vi "RTTAutomation.vi"() -> ()   [LabVIEW 2011]
doc: "This application is used to build test scripts for embedded software validation through the design process (MIL, HIL, TestCells)"
uses:
  SubVIs/TS_controls.ctl
  SubVIs/UI_Pages.ctl
  SubVIs/ScriptStepTypeDef.ctl
panel:
  in  "Stop":bool
  in  "Navigation Bar":T1
  in  "TestStand UI ExecutionView Manager":refnum<k7>(container)
  in  "TestStand UI SequenceFileView Manager":refnum<k7>(container)
  in  "Tab Control":T2(tab)
  out "State":string="Ready"
  out "Saved?":bool=TRUE
  in  "Save As Test Script":bool
  in  "Add_Test Procedure":bool
  in  "TreeCtl":string(tree)="System Config"
  in  "Open Test Script":bool
  in  "Save Test Script":bool
  in  "New Test Script":bool
  in  "Run Seq":refnum<k7>(container)
  in  "Open Seq file":refnum<k7>(container)
  in  "Test Sequence Viewer":refnum<k7>(container) caption="TestStand Sequence"
  in  "Generate":bool
  in  "Report Viewer":refnum<k7>(container)
  in  "Open DDreport":bool
  in  "Open TS Report":bool
  in  "Configuration Paths":T3
  out "Missing Files":bool
  in  "TestStand UI Application Manager (in)":refnum<k7>(container)
  # "Real-Time Test Automation"
  # "Test Script Builder"
  # "Sequence Builder"
  # "Report Viewer"
  # "Utilities"
  # "System Configuration"
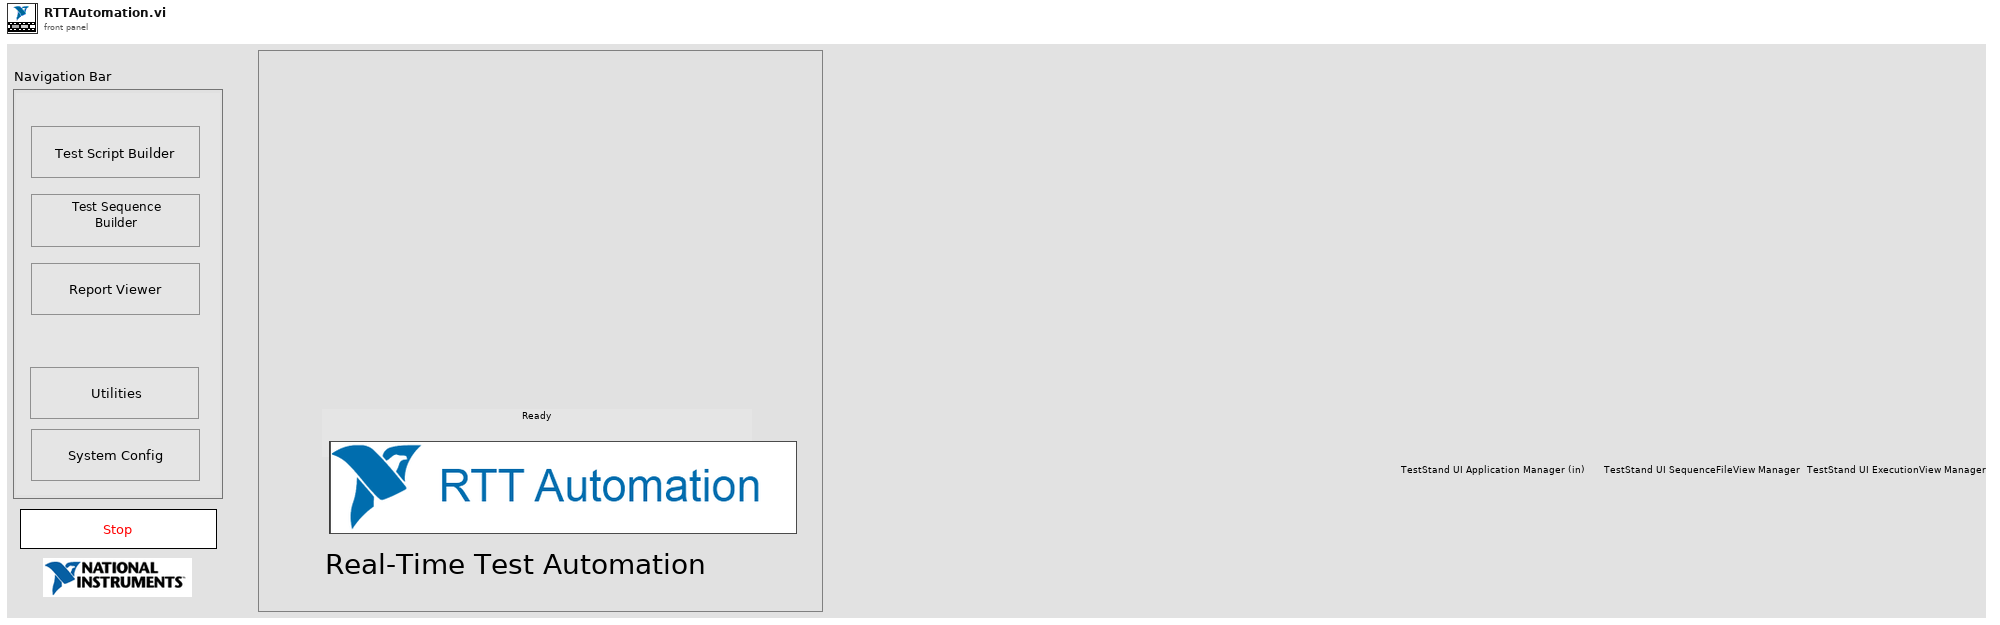
[diagram p1: front panel]
types:
  T1 = cluster{"Script Builder":bool, "Test Sequence Builder":bool, "Report":bool, "Utilities":bool, "System Config":bool}
  T2 = enum32{"Splash", "Test Script Builder", "Sequence Builder", "Report", "Utilities", "System Config"}
  T3 = cluster{"Working Directory":path, "Folder to Requirements Document":path, "Folder to the VeriStand Projects":path, "Folder to Stimuls Profiles":path, "Folder to Calibration files":path, "Folder to Analysis Scripts":path}
  T4 = typedef "ScriptStepTypeDef.ctl" = cluster{"Indent Level":i32, "Tag":string, "Step component":string, "Req":string, "Parent Tag":string, "Symbol Index":i32}
  T5 = enum8{"Enabled", "Disabled", "Disabled and Grayed Out"}
  T6 = typedef "UI_Pages.ctl" = enum32{"Splash", "Test Script Builder", "Sequence Builder", "Report", "Utilities", "System Config"}
  T7 = typedef "TS_controls.ctl" = cluster{"Open Seq file":refnum<k7>, "Test Sequence Viewer":refnum<k7>, "Run Seq":refnum<k7>}
  T8 = typedef "Config cluster.ctl" = cluster{"Working Directory":path, "Folder to Requirements Documents":path, "Folder to VeriStand Project files":path, "Folder to Stimuls Profiles":path, "Folder to Calibration files":path, "Folder to Analysis Scripts":path, "Requirements":string[], "Tree Control":refnum<vi>, "vi reference":refnum<vi>}
  T9 = typedef "LVPoint32TypeDef.ctl" = cluster{"Horizontal":i32, "Vertical":i32}
  T10 = enum32{"invalid app kind", "Development System", "Run Time System", "Student Edition", "Embedded LabVIEW", "Evaluation", "Custom"}
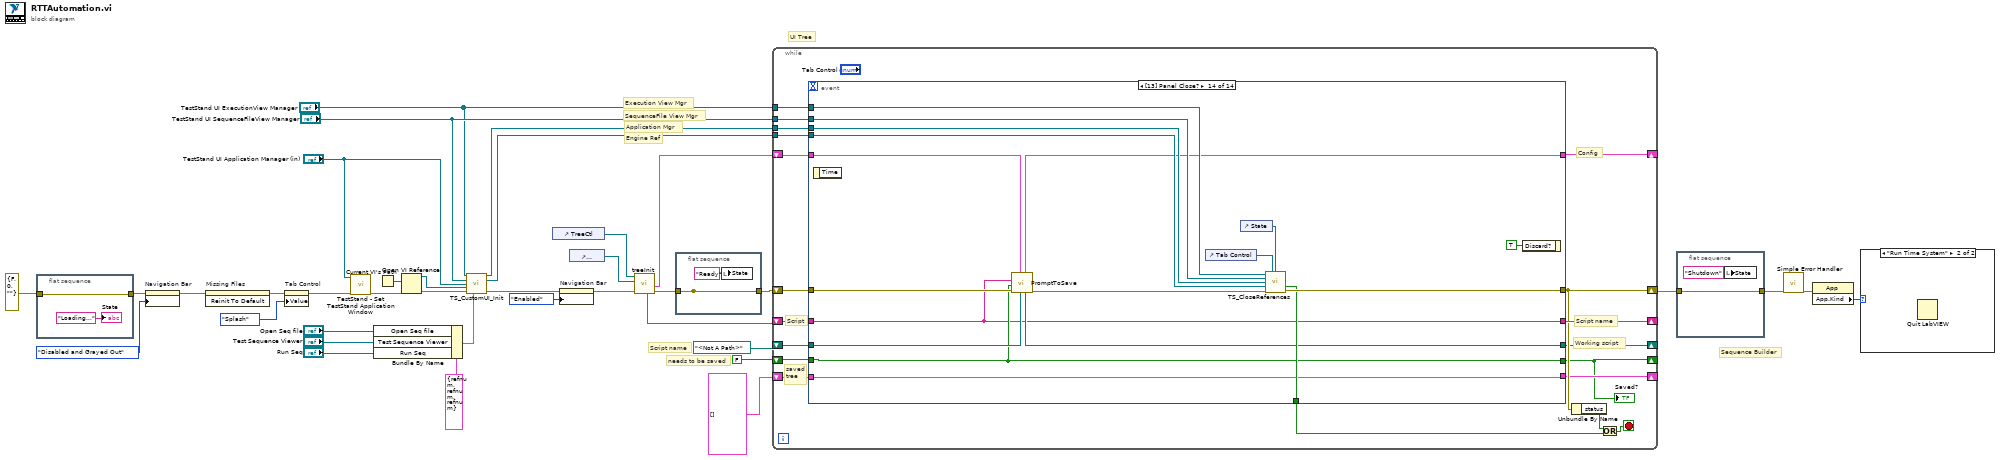
[diagram p0: block diagram]
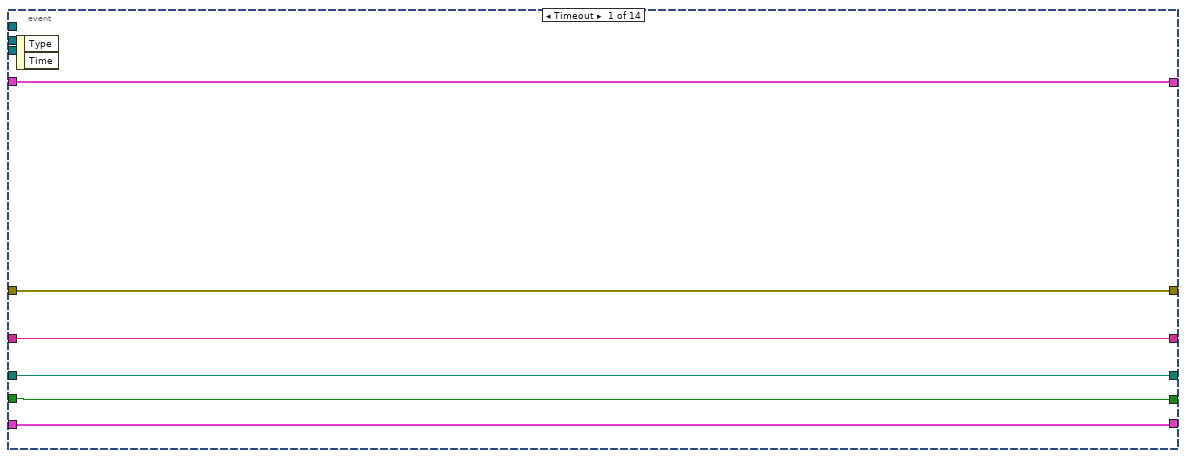
[diagram p3: hidden frame]
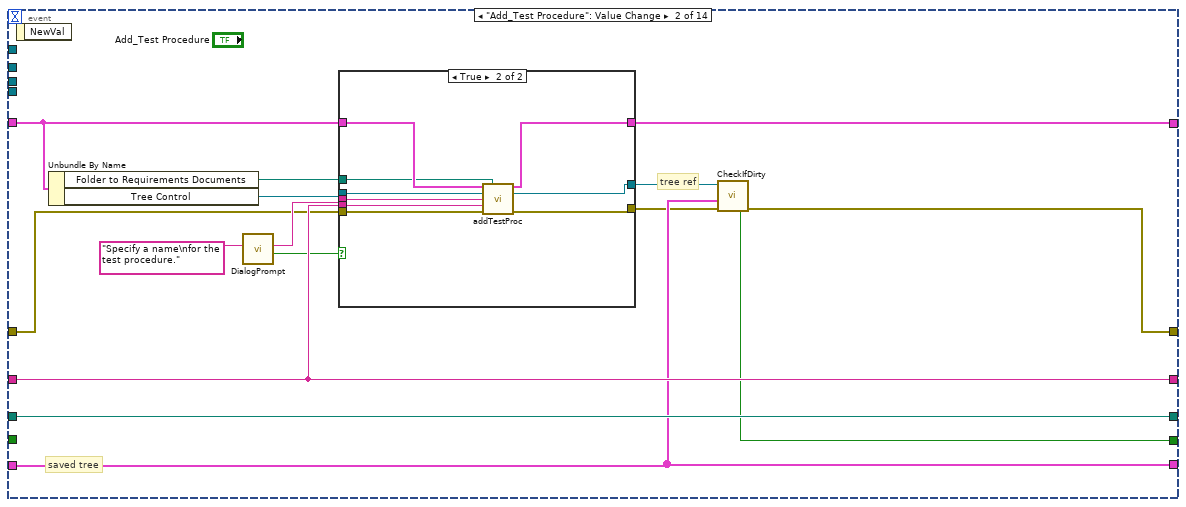
[diagram p4: hidden frame]
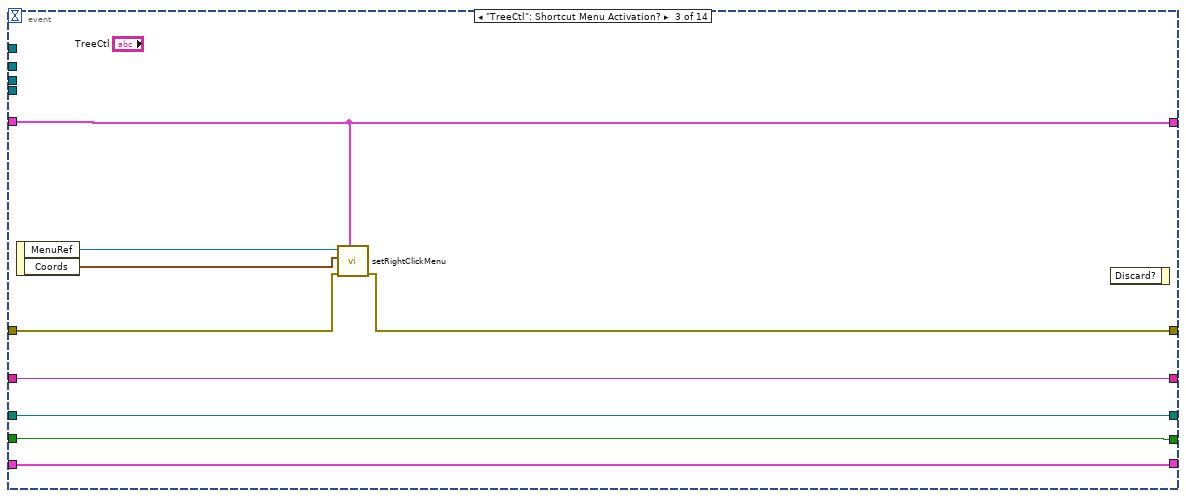
[diagram p6: hidden frame]
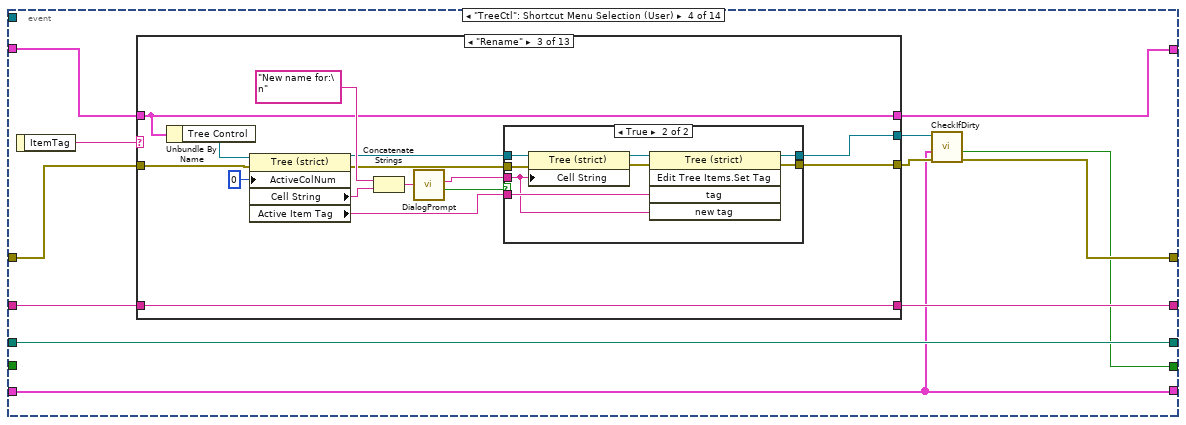
[diagram p7: hidden frame]
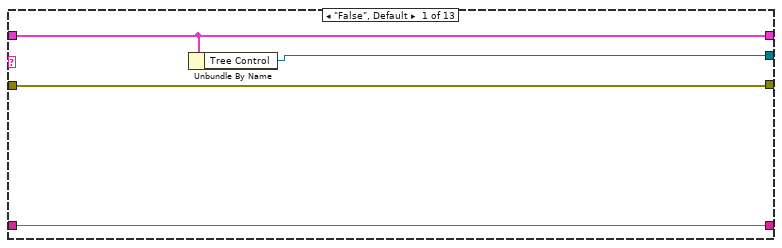
[diagram p8: hidden frame]
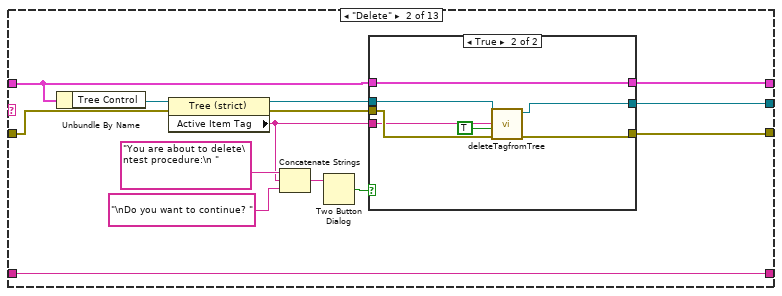
[diagram p9: hidden frame]
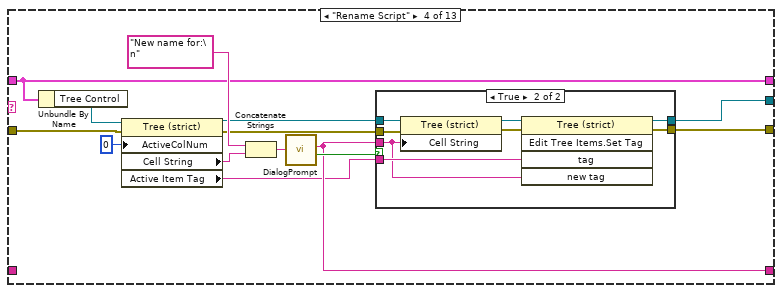
[diagram p12: hidden frame]
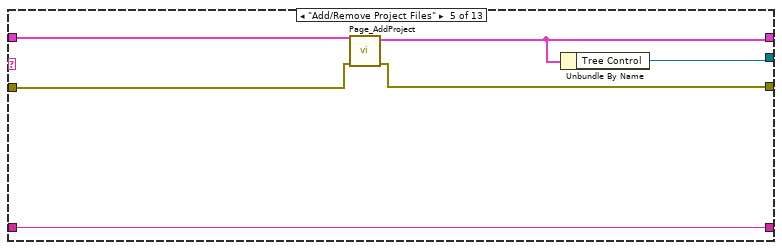
[diagram p14: hidden frame]
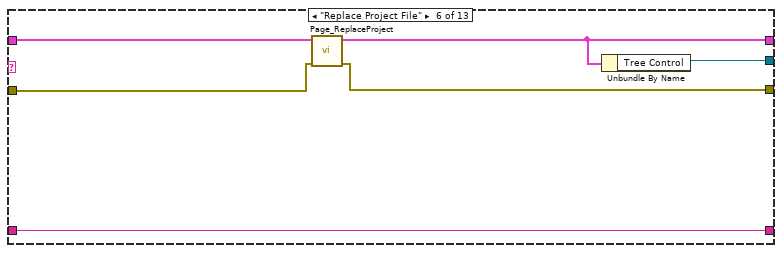
[diagram p15: hidden frame]
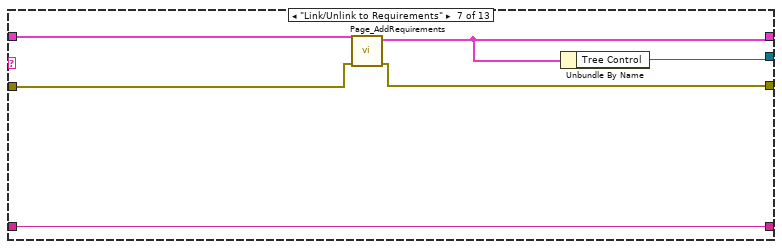
[diagram p16: hidden frame]
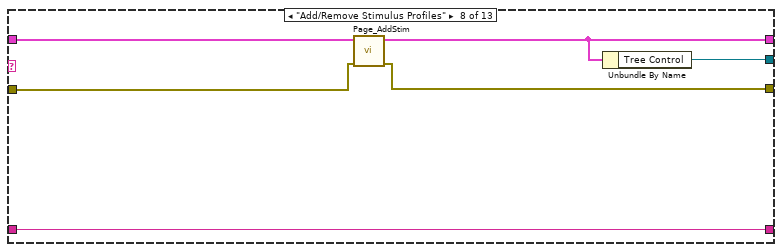
[diagram p17: hidden frame]
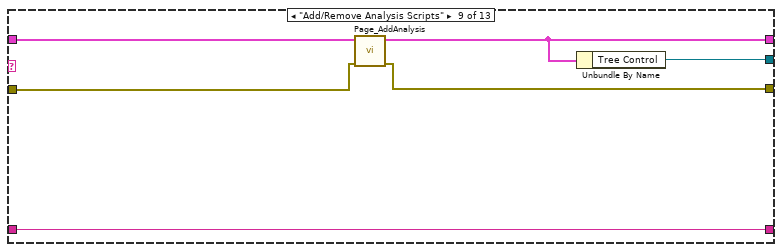
[diagram p18: hidden frame]
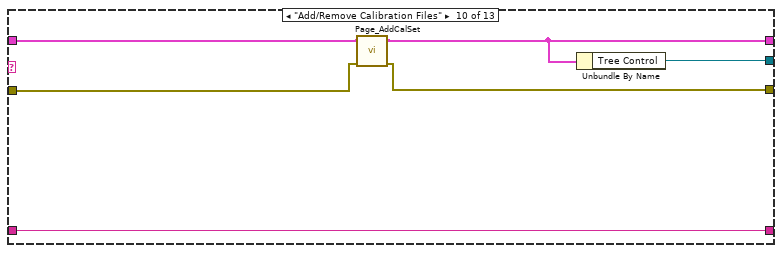
[diagram p19: hidden frame]
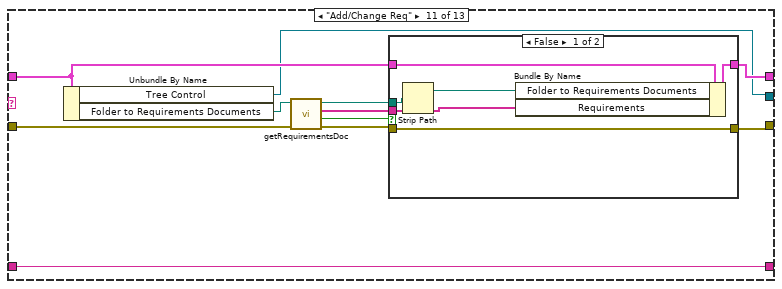
[diagram p20: hidden frame]
diagram:
  # "needs to be saved"
  # "Execution View Mgr"
  # "SequenceFile View Mgr"
  # "Engine Ref"
  # "Application Mgr"
  # "Script name"
  # "Sequence Builder"
  # "UI Tree"
  n1 = flat-sequence {
    tunnel: errorcluster {"status"=FALSE, "code"=0, "source"=""} ("error in (no error)") -> [w38]
    tunnel: [w38] -> w19
    frame #0 {
      "State" <- "Loading..." ("State")
    }
  }
  n2 = property on="Navigation Bar" class="Clust"(error in=w19, "DisabledEnum"=T5."Disabled and Grayed Out" ("Disabled")) -> (error out=w4:errorcluster)  [unwired: 1 in, 1 out]
  n3 = invoke on="Missing Files" class="Bool (strict)" method="Reinit To Default"(error in=w4) -> (error out=w5:errorcluster)  [unwired: 2 in, 2 out]
  n4 = property on="Tab Control" class="TabCtl (strict)"(error in=w5, "Value"=UI_Pages."Splash" ("UI Page")) -> (error out=w27:errorcluster)  [unwired: 1 in, 1 out]
  n5 = call <vilib>:"TestStand - Set TestStand Application Window.vi"("error in (no error)"=w27, "Application Manager"="TestStand UI Application Manager (in)") -> ("error out"=w26:errorcluster)  [unwired: 9 in]
  n6 = Bundle By Name(cluster=T7 {"Open Seq file"=refnum, "Test Sequence Viewer"=refnum, "Run Seq"=refnum} ("Controls"), "Open Seq file"="Open Seq file", "Test Sequence Viewer"="Test Sequence Viewer", "Run Seq"="Run Seq") -> (w8:T7)
  n7 = Current VI's Path() -> (path=w37:path)
  n8 = Open VI Reference(vi path=w37, error in (no error)=w26) -> (vi reference=w9:refnum<vi>, error out=w35:errorcluster)  [unwired: 4 in]
  n9 = call "TS_CustomUI_Init.vi"("TestStand UI ExecutionView Manager"="TestStand UI ExecutionView Manager", "TestStand UI SequenceFileView Manager"="TestStand UI SequenceFileView Manager", "TestStand UI Application Manager (in)"="TestStand UI Application Manager (in)", "VI Refnum"=w9, "error in"=w35, "Controls"=w8) -> ("TestStand UI Application Manager (out)"=w36:refnum<k7>, "Engine Ref out"=w13:refnum<k7>, "error out"=w24:errorcluster)  [unwired: 7 in]
  n10 = control-ref of="TreeCtl"() -> (w31:refnum<vi>)
  n11 = property on="Navigation Bar" class="Clust"(error in=w24, "DisabledEnum"=T5."Enabled" ("Disabled")) -> (error out=w23:errorcluster)  [unwired: 1 in, 1 out]
  n12 = control-ref of="Configuration Paths"() -> (w14:refnum<vi>)
  n13 = call "treeInit.vi"("error in"=w23, "Configuration Paths"=w14, "Tree Refnum"=w31) -> ("error out"=w16:errorcluster, "Config Cluster out"=w29:T8, "Script name"=w28:string)  [unwired: 6 in]
  n14 = flat-sequence {
    tunnel: [w40] -> _
    tunnel: [w40] -> w15
    tunnel: w16 -> [w40]
    frame #0 {
      n15 = local write "State"("Ready" ("State")) -> ()
    }
  }
  n16 = while {
    tunnel: w36 -> [w51]
    tunnel: "TestStand UI SequenceFileView Manager" -> [w60]
    shift-right: [w59] -> _
    shift-left: w29 -> [w58]
    shift-right: [w57] -> _
    shift-left: w28 -> [w56]
    shift-right: [w53] -> w18
    shift-left: w15 -> [w55]
    tunnel: "TestStand UI ExecutionView Manager" -> [w50]
    shift-right: [w48] -> _
    shift-left: path "<Not A Path>" ("selected path") -> [w49]
    tunnel: w13 -> [w47]
    shift-right: [w45] -> _
    shift-left: T4[] [] ("Steps with Params") -> [w44]
    shift-right: [w43] -> _
    shift-left: FALSE -> [w42]
    stop <- w54 stop-if-true
    # "saved\ntree"
    # "Working script"
    # "Script"
    # "Config"
    # "Script name"
    n17 = event shown="[13] Panel Close?" {
      selector: _ -> [_ _ _ _ _ _ _ _ _ _ _ _ _ _]
      dyn-events: _ -> [_ _ _ _ _ _ _ _ _ _ _ _ _ _]
      timeout: _ -> [_ _ _ _ _ _ _ _ _ _ _ _ _ _]
      tunnel: [w65 w68 w94 w105 w284 w299 w321 w331 w338 w366 w388 w418 w435 w453] -> w53
      tunnel: w51 -> [_ _ _ _ _ _ w323 _ _ _ _ _ w432 w450]
      tunnel: w60 -> [_ _ _ _ _ _ _ _ _ _ _ _ w433 w451]
      tunnel: [w66 w74 w98 w112 w282 w302 w314 w324 w347 w368 w393 w420 w426 w444] -> w59
      tunnel: w58 -> [w66 w75 w98 w113 w287 w302 w315 w324 w347 w368 w392 w420 w425 w443]
      tunnel: [w64 w79 w102 w111 w289 w307 w317 w330 w352 w373 w395 w419 w421 w439] -> w57
      tunnel: w56 -> [w64 w79 w102 w110 w289 w307 w317 w329 w352 w377 w396 w419 w421 w439]
      tunnel: w55 -> [w65 w78 w95 w109 w285 w304 w319 w332 w348 w376 w399 w418 w428 w446]
      tunnel: w50 -> [_ _ _ _ _ _ _ _ _ _ _ _ w434 w452]
      tunnel: w49 -> [w63 w77 w101 w108 w288 w306 w313 w328 w336 w375 w391 w412 w423 w441]
      tunnel: [w63 w77 w101 w108 w288 w306 w312 w327 w336 w374 w394 w412 w424 w442] -> w48
      tunnel: w47 -> [_ _ _ _ _ _ w322 _ _ _ _ _ w431 w449]
      tunnel: [_ _ _ _ _ _ _ _ _ _ _ _ w430 w448] -> w46
      tunnel: [w62 w72 w100 w104 w283 w303 w320 w325 w334 w369 w383 w410 w429 w447] -> w45
      tunnel: w44 -> [w62 w72 w100 w104 w283 w303 w320 w326 w334 w372 w384 w410 w429 w447]
      tunnel: [w61 w70 w99 w103 w286 w305 w316 TRUE w335 w371 w385 w411 w422 w440] -> w43
      tunnel: w42 -> [w61 _ w99 _ w286 w305 w316 _ w335 _ w386 w411 w422 w440]
      event Timeout {
        n18 = event-data() -> ()  [unwired: 1 in, 2 out]
      }
      event "Add_Test Procedure": Value Change {
        # "saved tree"
        # "tree ref"
        n19 = event-data() -> ()  [unwired: 1 in, 1 out]
        n20 = Unbundle By Name(w75) -> ("Folder to Requirements Documents"=w76:path, "Tree Control"=w71:refnum<vi>)
        n21 = call "DialogPrompt.vi"("Dialog prompt"="Specify a name\nfor the test procedure.") -> ("OK out"=w73:bool, "Usert Txt(out)"=w81:string)  [unwired: 9 in]
        n22 = case shown="True" w73 {
          tunnel: w71 -> [w82 w90]
          tunnel: w81 -> [_ w89]
          tunnel: w79 -> [_ w88]
          tunnel: w78 -> [w84 w87]
          tunnel: [w84 w86] -> w69
          tunnel: w76 -> [_ w91]
          tunnel: w75 -> [w83 w93]
          tunnel: [w83 w92] -> w74
          tunnel: [w82 w85] -> w67
          frame False {
          }
          frame True {
            n23 = call "addTestProc.vi"("Config Cluster"=w93, "Tree Control"=w90, "Procedure name"=w89, "Script name"=w88, "error in"=w87, "Folder to Requirements Documents"=w91) -> ("Config Cluster out"=w92:T8, "Tree Control out"=w85:refnum<vi>, "error out"=w86:errorcluster)  [unwired: 7 in]
          }
        }
        n24 = call "CheckIfDirty.vi"("error in"=w69, "Saved Tree"=w72, "Tree Control"=w67) -> ("error out"=w68:errorcluster, "Dirty Flag"=w70:bool)  [unwired: 6 in, 1 out]
      }
      event "TreeCtl": Shortcut Menu Activation? {
        n25 = event-data() -> ("MenuRef"=w96:refnum<k9>, "Coords"=w97:T9)  [unwired: 1 in]
        n26 = call "setRightClickMenu.vi"("Config Cluster"=w98, "error in"=w95, "Coords"=w97, "MenuRef"=w96) -> ("error out"=w94:errorcluster)  [unwired: 7 in]
        n27 = event-data() -> ()  [unwired: 2 in, 1 out]
      }
      event "TreeCtl": Shortcut Menu Selection (User) {
        n28 = event-data() -> ("ItemTag"=w114:string)  [unwired: 1 in]
        n29 = case shown="\"Rename\"" w114 {
          tunnel: w113 -> [w116 w125 w151 w175 w197 w203 w207 w215 w221 w226 w235 w259 w269]
          tunnel: [w116 w127 w151 w175 w194 w200 w206 w212 w218 w225 w229 w259 w269] -> w112
          tunnel: [w118 w132 w143 w173 w192 w198 w208 w210 w216 w222 w238 w256 w267] -> w111
          tunnel: w110 -> [w118 w132 w143 _ w192 w198 w208 w210 w216 w222 w238 w256 w267]
          tunnel: w109 -> [w117 w124 w148 w172 w196 w201 w205 w214 w219 w224 w236 w248 w262]
          tunnel: [w117 w126 w146 w170 w195 w202 w204 w213 w220 w223 w230 w250 w264] -> w106
          tunnel: [w115 w119 w144 w168 w193 w199 w209 w211 w217 w227 w228 w247 w261] -> w107
          frame "False", Default {
            n30 = Unbundle By Name(w116) -> ("Tree Control"=w115:refnum<vi>)
          }
          frame "Delete" {
            n31 = Unbundle By Name(w125) -> ("Tree Control"=w122:refnum<vi>)
            n32 = property class="Tree (strict)"(reference=w122, error in=w124) -> (reference out=w121:refnum<vi>, error out=w123:errorcluster, "Active Item Tag"=w120:string)
            n33 = Concatenate Strings("You are about to delete\ntest procedure:\n ", w120, "\nDo you want to continue? " ("string")) -> (w129:string)
            n34 = Two Button Dialog(message=w129) -> (T button?=w128:bool)  [unwired: 2 in]
            n35 = case shown="True" w128 {
              tunnel: w125 -> [w135 w139]
              tunnel: [w135 w139] -> w127
              tunnel: w123 -> [w134 w142]
              tunnel: [w134 w141] -> w126
              tunnel: w121 -> [w133 w138]
              tunnel: w120 -> [_ w137]
              tunnel: [w133 w136] -> w119
              frame False {
              }
              frame True {
                n36 = call "deleteTagfromTree.vi"("error in (no error)"=w142, "Delete Children?"=TRUE, "Tag"=w137, "Tree Ref"=w138) -> ("error out"=w141:errorcluster, "Tree ref out"=w136:refnum<vi>)  [unwired: 6 in]
              }
            }
          }
          frame "Rename" {
            n37 = Unbundle By Name(w151) -> ("Tree Control"=w150:refnum<vi>)
            n38 = property class="Tree (strict)"(reference=w150, error in=w148, "ActiveColNum"=0 ("Active Cell:Active Column Number")) -> (reference out=w153:refnum<vi>, error out=w147:errorcluster, "Cell String"=w154:string, "Active Item Tag"=w145:string)
            n39 = Concatenate Strings("New name for:\n" ("Dialog prompt"), w154) -> (w156:string)
            n40 = call "DialogPrompt.vi"("Dialog prompt"=w156) -> ("OK out"=w152:bool, "Usert Txt(out)"=w149:string)  [unwired: 9 in]
            n41 = case shown="True" w152 {
              tunnel: w149 -> [_ w161]
              tunnel: w153 -> [w158 w167]
              tunnel: w147 -> [w159 w166]
              tunnel: [w159 w163] -> w146
              tunnel: w145 -> [_ w162]
              tunnel: [w158 w160] -> w144
              frame False {
              }
              frame True {
                n42 = property class="Tree (strict)"(reference=w167, error in=w166, "Cell String"=w161) -> (reference out=w165:refnum<vi>, error out=w164:errorcluster)
                n43 = invoke class="Tree (strict)" method="Edit Tree Items.Set Tag"(reference=w165, error in=w164, "tag"=w162, "new tag"=w161) -> (reference out=w160:refnum<vi>, error out=w163:errorcluster)  [unwired: 1 in, 3 out]
              }
            }
          }
          frame "Rename Script" {
            n44 = Unbundle By Name(w175) -> ("Tree Control"=w174:refnum<vi>)
            n45 = property class="Tree (strict)"(reference=w174, error in=w172, "ActiveColNum"=0 ("Active Cell:Active Column Number")) -> (reference out=w177:refnum<vi>, error out=w171:errorcluster, "Cell String"=w178:string, "Active Item Tag"=w169:string)
            n46 = Concatenate Strings("New name for:\n" ("Dialog prompt"), w178) -> (w180:string)
            n47 = call "DialogPrompt.vi"("Dialog prompt"=w180) -> ("OK out"=w176:bool, "Usert Txt(out)"=w173:string)  [unwired: 9 in]
            n48 = case shown="True" w176 {
              tunnel: w173 -> [_ w185]
              tunnel: w177 -> [w182 w191]
              tunnel: w171 -> [w183 w190]
              tunnel: [w183 w187] -> w170
              tunnel: w169 -> [_ w186]
              tunnel: [w182 w184] -> w168
              frame False {
              }
              frame True {
                n49 = property class="Tree (strict)"(reference=w191, error in=w190, "Cell String"=w185) -> (reference out=w189:refnum<vi>, error out=w188:errorcluster)
                n50 = invoke class="Tree (strict)" method="Edit Tree Items.Set Tag"(reference=w189, error in=w188, "tag"=w186, "new tag"=w185) -> (reference out=w184:refnum<vi>, error out=w187:errorcluster)  [unwired: 1 in, 3 out]
              }
            }
          }
          frame "Add/Remove Project Files" {
            n51 = call "Page_AddProject.vi"("error in (no error)"=w196, "Configuration Paths in"=w197) -> ("error out"=w195:errorcluster, "Configuration Paths out"=w194:T8)  [unwired: 8 in]
            n52 = Unbundle By Name(w194) -> ("Tree Control"=w193:refnum<vi>)
          }
          frame "Replace Project File" {
            n53 = call "Page_ReplaceProject.vi"("error in (no error)"=w201, "Configuration Paths in"=w203) -> ("error out"=w202:errorcluster, "Configuration Paths out"=w200:T8)  [unwired: 8 in]
            n54 = Unbundle By Name(w200) -> ("Tree Control"=w199:refnum<vi>)
          }
          frame "Link/Unlink to Requirements" {
            n55 = call "Page_AddRequirements.vi"("error in (no error)"=w205, "Configuration Paths"=w207) -> ("error out"=w204:errorcluster, "Configuration Paths out"=w206:T8)  [unwired: 8 in]
            n56 = Unbundle By Name(w206) -> ("Tree Control"=w209:refnum<vi>)
          }
          frame "Add/Remove Stimulus Profiles" {
            n57 = call "Page_AddStim.vi"("error in (no error)"=w214, "Configuration Paths"=w215) -> ("error out"=w213:errorcluster, "Configuration Paths out"=w212:T8)  [unwired: 8 in]
            n58 = Unbundle By Name(w212) -> ("Tree Control"=w211:refnum<vi>)
          }
          frame "Add/Remove Analysis Scripts" {
            n59 = call "Page_AddAnalysis.vi"("error in (no error)"=w219, "Configuration Paths"=w221) -> ("error out"=w220:errorcluster, "Configuration Paths out"=w218:T8)  [unwired: 8 in]
            n60 = Unbundle By Name(w218) -> ("Tree Control"=w217:refnum<vi>)
          }
          frame "Add/Remove Calibration Files" {
            n61 = call "Page_AddCalSet.vi"("error in (no error)"=w224, "Configuration Paths"=w226) -> ("error out"=w223:errorcluster, "Configuration Paths out"=w225:T8)  [unwired: 8 in]
            n62 = Unbundle By Name(w225) -> ("Tree Control"=w227:refnum<vi>)
          }
          frame "Add/Change Req" {
            n63 = Unbundle By Name(w235) -> ("Tree Control"=w228:refnum<vi>, "Folder to Requirements Documents"=w237:path)
            n64 = call "getRequirementsDoc.vi"("error in (no error)"=w236, "Path"=w237) -> ("error out"=w231:errorcluster, "Cancelled?"=w232:bool, "Requirements"=w233:string[], "Req Doc Folder"=w234:path)  [unwired: 6 in]
            n65 = case shown="False" w232 {
              tunnel: w235 -> [w244 w246]
              tunnel: [w241 errorcluster {"status"=FALSE, "code"=0, "source"=""} ("error out")] -> w230
              tunnel: [w242 w246] -> w229
              tunnel: w231 -> [w241 _]
              tunnel: w233 -> [w240 _]
              tunnel: w234 -> [w239 _]
              frame False {
                n66 = Strip Path(path=w239) -> (stripped path=w243:path)  [unwired: 1 out]
                n67 = Bundle By Name(cluster=w244, "Folder to Requirements Documents"=w243, "Requirements"=w240) -> (w242:T8)
              }
              frame True {
              }
            }
          }
          frame "Conditional Run", "Unconditional Run" {
            w252 = 20 ("y")
            n68 = Unbundle By Name(w259) -> ("Tree Control"=w258:refnum<vi>)
            n69 = property class="Tree (strict)"(reference=w258, error in=w248) -> (reference out=w255:refnum<vi>, error out=w249:errorcluster, "Glyph"=w257:i32)
            n70 = Equal?(x=w257, y=w252) -> (x = y?=w254:bool)
            n71 = Select(t=120 ("y"), s=w254, f=w252) -> (s? t:f=w251:i32)
            n72 = property class="Tree (strict)"(reference=w255, error in=w249, "Glyph"=w251) -> (reference out=w247:refnum<vi>, error out=w250:errorcluster)
          }
          frame "Attended Run", "Unattended Run" {
            n73 = Unbundle By Name(w269) -> ("Tree Control"=w268:refnum<vi>)
            n74 = property class="Tree (strict)"(reference=w268, error in=w262) -> (reference out=w266:refnum<vi>, error out=w263:errorcluster, "Glyph"=w260:i32)
            n75 = case shown="10, 110" w260 {
              selector: w260 -> [w270 w271 w276]
              tunnel: [w270 w272 w277] -> w265
              frame 0, Default {
              }
              frame 30, 130 {
                w273 = 30 ("y")
                n76 = Equal?(x=w271, y=w273) -> (x = y?=w275:bool)
                n77 = Select(t=130 ("y"), s=w275, f=w273) -> (s? t:f=w272:i32)
              }
              frame 10, 110 {
                w278 = 10 ("y")
                n78 = Equal?(x=w276, y=w278) -> (x = y?=w280:bool)
                n79 = Select(t=110 ("y"), s=w280, f=w278) -> (s? t:f=w277:i32)
              }
            }
            n80 = property class="Tree (strict)"(reference=w266, error in=w263, "Glyph"=w265) -> (reference out=w261:refnum<vi>, error out=w264:errorcluster)
          }
        }
        n81 = call "CheckIfDirty.vi"("error in"=w106, "Saved Tree"=w104, "Tree Control"=w107) -> ("error out"=w105:errorcluster, "Dirty Flag"=w103:bool)  [unwired: 6 in, 1 out]
      }
      event "Configuration Paths": Value Change {
        n82 = event-data() -> ()  [unwired: 1 in, 1 out]
        n83 = Unbundle By Name("Configuration Paths") -> ("Working Directory"=w295:path, "Folder to Requirements Document"=w294:path, "Folder to Stimuls Profiles"=w293:path, "Folder to Calibration files"=w292:path, "Folder to Analysis Scripts"=w291:path, "Folder to the VeriStand Projects"=w290:path)
        n84 = Bundle By Name(cluster=w287, "Working Directory"=w295, "Folder to Requirements Documents"=w294, "Folder to Stimuls Profiles"=w293, "Folder to Calibration files"=w292, "Folder to Analysis Scripts"=w291, "Folder to VeriStand Project files"=w290) -> (w282:T8)
        n85 = control-ref of="Missing Files"() -> (w281:refnum<vi>)
        n86 = call "checkIfFilesExist.vi"("Saved Tree"=w283, "Config Cluster out"=w282, "error in (no error)"=w285, "Missing Files"=w281) -> ("error out"=w284:errorcluster)  [unwired: 5 in, 2 out]
      }
      event "Missing Files": Mouse Down {
        n87 = event-data() -> ()  [unwired: 1 in, 1 out]
        n88 = control-ref of="Missing Files"() -> (w297:refnum<vi>)
        n89 = call "checkIfFilesExist.vi"("Saved Tree"=w303, "Config Cluster out"=w302, "error in (no error)"=w304, "Missing Files"=w297) -> ("error out"=w300:errorcluster, "Files missing"=w301:bool, "Missing Files"=w298:string[])  [unwired: 5 in]
        n90 = case shown="True" w301 {
          tunnel: [w308 w311] -> w299
          tunnel: w300 -> [w308 w310]
          tunnel: w298 -> [_ w309]
          frame False {
          }
          frame True {
            n91 = call "Page_MissingFiles.vi"("error in"=w310, "Missing Files"=w309) -> ("error out"=w311:errorcluster)  [unwired: 9 in]
          }
        }
      }
      event "Generate": Value Change {
        n92 = event-data() -> ()  [unwired: 1 in, 1 out]
        n93 = call "PromptToSave.vi"("Working script"=w313, "Config Cluster in"=w315, "error in"=w319, "Script Saved?"=w316, "Script name"=w317) -> ("error out"=w318:errorcluster, "Working Script out"=w312:path, "Config Cluster out"=w314:T8)  [unwired: 4 in]
        n94 = call "SeqBuilder.vi"("Config Cluster"=w314, "error in"=w318, "Script name"=w317, "Engine Ref out"=w322, "TestStand UI Application Manager (out)"=w323) -> ("error out"=w321:errorcluster)  [unwired: 6 in]
      }
      event "New Test Script": Value Change {
        n95 = event-data() -> ()  [unwired: 1 in, 1 out]
        n96 = call "Script_New.vi"("Script name"=w329, "error in"=w332, "Working Script"=w328, "Saved Tree"=w326, "Config Cluster"=w324) -> ("Saved Tree out"=w325:T4[], "Working Script out"=w327:path, "Script name out"=w330:string, "error out"=w331:errorcluster)  [unwired: 11 in]
      }
      event "Open TS Report", "Open DDreport": Value Change {
        n97 = event-data() -> ("CtlRef"=w351:refnum<vi>)  [unwired: 1 in]
        n98 = property class="Bool"(reference=w351, error in=w348) -> (error out=w349:errorcluster, "Label.Text"=w345:string)  [unwired: 1 out]
        n99 = Unbundle By Name(w347) -> ("Working Directory"=w346:path)
        n100 = Equal?(x=w345, y="Open TS Report") -> (x = y?=w343:bool)
        n101 = Select(t="*.xml" ("y"), s=w343, f="*.htm" ("y")) -> (s? t:f=w342:string)
        n102 = call "File Dialog3"("start path"=w346, "error in"=w349, "pattern (all files)"=w342) -> ("selected path"=w339:path, "cancelled"=w337:bool, "error out"=w350:errorcluster)  [unwired: 9 in, 1 out]
        n103 = case shown="True" w337 {
          tunnel: w350 -> [w360 _]
          tunnel: w339 -> [w357 _]
          tunnel: [w353 errorcluster {"status"=FALSE, "code"=0, "source"=""} ("error out")] -> w338
          frame False {
            n104 = Path To String(path=w357) -> (string=w356:string)
            n105 = Automation Open(error in (no error)=w360, Automation Refnum="Report Viewer") -> (Automation Refnum=w359:refnum<k7>, error out=w358:errorcluster)  [unwired: 2 in]
            n106 = invoke class="IWebBrowser2" method="Navigate"(reference=w359, error in=w358, "URL"=w356) -> (reference out=w355:refnum<k7>, error out=w354:errorcluster)  [unwired: 5 in, 6 out]
            n107 = Close Reference(reference=w355, error in (no error)=w354) -> (error out=w353:errorcluster)
          }
          frame True {
          }
        }
      }
      event "Open Test Script": Value Change {
        n108 = event-data() -> ()  [unwired: 1 in, 1 out]
        n109 = call "Script_Open.vi"("Script name"=w377, "error in"=w376, "Working script"=w375, "Saved Tree"=w372, "Config Cluster"=w368) -> ("Saved tree out"=w369:T4[], "Working script out"=w374:path, "Script name out"=w373:string, "Dirty Flag"=w371:bool, "error out"=w370:errorcluster)  [unwired: 10 in]
        n110 = control-ref of="Missing Files"() -> (w363:refnum<vi>)
        n111 = call "checkIfFilesExist.vi"("Saved Tree"=w369, "Config Cluster out"=w368, "error in (no error)"=w370, "Missing Files"=w363) -> ("error out"=w367:errorcluster, "Files missing"=w364:bool, "Missing Files"=w365:string[])  [unwired: 5 in]
        n112 = case shown="True" w364 {
          tunnel: w367 -> [w378 w381]
          tunnel: [w378 w380] -> w366
          tunnel: w365 -> [_ w379]
          frame False {
          }
          frame True {
            n113 = call "Page_MissingFiles.vi"("error in"=w381, "Missing Files"=w379) -> ("error out"=w380:errorcluster)  [unwired: 9 in]
          }
        }
      }
      event "Save Test Script", "Save As Test Script": Value Change {
        # "current tree"
        n114 = event-data() -> ("CtlRef"=w405:refnum<vi>)  [unwired: 1 in]
        n115 = property class="Bool"(reference=w405, error in=w399) -> (error out=w398:errorcluster, "Label.Text"=w403:string)  [unwired: 1 out]
        n116 = Not Equal?(x=path "<Not A Path>" ("selected path"), y=w391) -> (x != y?=w400:bool)
        n117 = Equal?(x=w403, y="Save Test Script") -> (x = y?=w402:bool)
        n118 = And(x=w402, y=w400) -> (x .and. y?=w397:bool)
        n119 = call "Script_Save.vi"("Config Cluster in"=w392, "Save/SaveAs(Save= True)"=w397, "Script name"=w396, "error in"=w398, "Working Script"=w391) -> ("Config Cluster out"=w393:T8, "Tree Control out"=w389:refnum<vi>, "Cancelled"=w387:bool, "Script name out"=w395:string, "Working Script out"=w394:path, "error out"=w390:errorcluster)  [unwired: 5 in]
        n120 = call "CheckIfDirty.vi"("error in"=w390, "Tree Control"=w389) -> ("error out"=w388:errorcluster, "Current Tree"=w382:T4[])  [unwired: 7 in, 1 out]
        n121 = case shown="True" w387 {
          tunnel: w386 -> [_ w409]
          tunnel: [FALSE w409] -> w385
          tunnel: w384 -> [_ w408]
          tunnel: [w406 w408] -> w383
          tunnel: w382 -> [w406 _]
          frame False {
          }
          frame True {
          }
        }
      }
      event "Navigation Bar": Value Change {
        n122 = event-data() -> ()  [unwired: 1 in, 1 out]
        n123 = Cluster To Array(cluster="Navigation Bar") -> (array=w416:bool[])
        n124 = Search 1D Array(1D array=w416, element=TRUE) -> (index of element=w414:i32)  [unwired: 1 in]
        n125 = Increment(x=w414) -> (x+1=w413:i32)
        n126 = property on="Tab Control" class="TabCtl (strict)"("Value"=w413) -> ()  [unwired: 2 in, 2 out]
      }
      event "Stop": Value Change {
        n127 = event-data() -> ()  [unwired: 1 in, 1 out]
        n128 = call "PromptToSave.vi"("Working script"=w423, "Config Cluster in"=w425, "error in"=w428, "Script Saved?"=w422, "Script name"=w421) -> ("error out"=w427:errorcluster, "Working Script out"=w424:path, "Config Cluster out"=w426:T8)  [unwired: 4 in]
        n129 = control-ref of="Tab Control"() -> (w437:refnum<vi>)
        n130 = control-ref of="State"() -> (w436:refnum<vi>)
        n131 = call "TS_CloseReferences.vi"("TestStand UI ExecutionView Manager"=w434, "TabCtl Refnum"=w437, "Str Refnum"=w436, "TestStand UI SequenceFileView Manager"=w433, "TestStand UI Application Manager (in)"=w432, "Engine Ref in"=w431, "error in"=w427) -> ("Shutdown"=w430:bool, "error out"=w435:errorcluster)  [unwired: 7 in]
      }
      event Panel Close? {
        n132 = event-data() -> ()  [unwired: 1 in, 1 out]
        n133 = call "PromptToSave.vi"("Working script"=w441, "Config Cluster in"=w443, "error in"=w446, "Script Saved?"=w440, "Script name"=w439) -> ("error out"=w445:errorcluster, "Working Script out"=w442:path, "Config Cluster out"=w444:T8)  [unwired: 4 in]
        n134 = control-ref of="Tab Control"() -> (w455:refnum<vi>)
        n135 = control-ref of="State"() -> (w454:refnum<vi>)
        n136 = call "TS_CloseReferences.vi"("TestStand UI ExecutionView Manager"=w452, "TabCtl Refnum"=w455, "Str Refnum"=w454, "TestStand UI SequenceFileView Manager"=w451, "TestStand UI Application Manager (in)"=w450, "Engine Ref in"=w449, "error in"=w445) -> ("Shutdown"=w448:bool, "error out"=w453:errorcluster)  [unwired: 7 in]
        n137 = event-data("Discard?"=TRUE) -> ()  [unwired: 1 in, 1 out]
      }
    }
    "Saved?" <- w43
    n138 = Unbundle By Name(w53) -> ("status"=w52:bool)
    n139 = Or(x=w52, y=w46) -> (x .or. y?=w54:bool)
  }
  n140 = flat-sequence {
    tunnel: w18 -> [w457]
    tunnel: [w457] -> w3
    frame #0 {
      n141 = local write "State"("Shutdown" ("State")) -> ()
    }
  }
  n142 = call <vilib>:"Simple Error Handler.vi"("error in (no error)"=w3) -> ("error out"=w2:errorcluster)  [unwired: 4 in, 4 out]
  n143 = property class="App"(error in=w2) -> ("App.Kind"=w1:T10)  [unwired: 1 in, 2 out]
  n144 = case shown="\"Run Time System\"" w1 {
    frame Default {
    }
    frame "Run Time System" {
      n145 = Quit LabVIEW() -> ()  [unwired: 1 in]
    }
  }
